vi "Get CaseFrame Index By CaseName.vi"(8 "error in (no error)":errorcluster, 10 "CASE":string, 11 "CSM-Helper in":refnum<class "CSM-Helper.lvclass">) -> (0 "error out":errorcluster, 1 "CaseStruRef":refnum<vi>, 2 "index":i32, 3 "CSM-Helper out":refnum<class "CSM-Helper.lvclass">)   [LabVIEW 2017, in "CSM-Helper.lvclass"]
doc: "### Get CaseFrame Index By CaseName.vi\n\n-- <b>Controls</b> --\n- <b>CASE</b>:\n- <b>CSM-Helper in</b>: CSMHelper input\n\n-- <b>Indicators</b> --\n- <b>index</b>:\n- <b>CSM-Helper out</b>: CSMHelper output"
uses:
  CSM-Helper.lvclass
  CSM-Helper.lvclass/CSM-Helper.ctl
  Properties/Read Case Structure Ref.vi
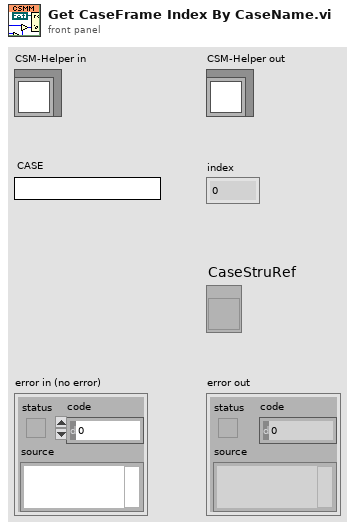
[diagram p1: front panel]
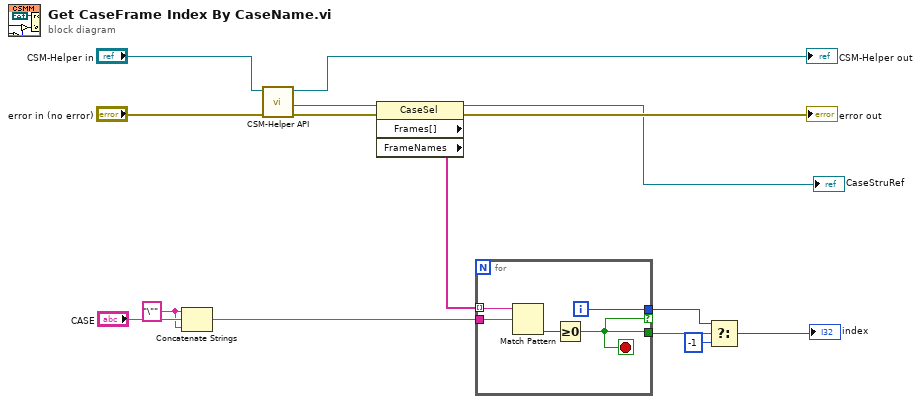
[diagram p0: block diagram]
diagram:
  w12 = "\"" ("string")
  n1 = Concatenate Strings(w12, "CASE", w12) -> (w13:string)
  n2 = call-poly "CSM-Helper API.vi"("error in (no error)"="error in (no error)", "CSM-Helper in"="CSM-Helper in") -> ("error out"=w7:errorcluster, "Case Structure"=w8:refnum<vi>, "CSM-Helper out"=→"CSM-Helper out":refnum<class "CSM-Helper.lvclass">)  [unwired: 7 in]
  n3 = property class="CaseSel" props=["Frames[]", "FrameNames"](reference=w8, error in=w7) -> (reference out=→"CaseStruRef":refnum<vi>, error out=→"error out":errorcluster, "FrameNames"=w15:string[])  [unwired: 1 out]
  n4 = for {
    tunnel: w15 -> [w20] mode=indexing
    tunnel: w13 -> [w19]
    tunnel: [w18] -> w4 if=w16
    tunnel: [w16] -> w5
    i -> [w18]
    stop <- w16 stop-if-true
    n5 = Match Pattern(string=w20, regular expression=w19) -> (offset past match=w17:i32)  [unwired: 1 in, 3 out]
    n6 = Greater Or Equal To 0?(x=w17) -> (x >= 0?=w16:bool)
  }
  n7 = Select(t=w4, s=w5, f=-1) -> (s? t:f=→"index":i32)
